vi "Initialize Battle Dialog.vi"() -> (2 "Dashboard":T1[](array[typedef]), 3 "SquareBattle out":refnum<class "SquareBattle Arena.lvclass">, 4 "Intensity Graph Values":cluster{dbl, u32}[](array[cluster]), 6 "Continue?":bool)   [LabVIEW 2014, in "SquareBattle Arena.lvlib" / "SquareBattle Arena.lvclass"]
uses:
  SquareBattle Arena.lvclass
  Dashboard.ctl
  Runner Cluster.ctl
  Square/Square.lvclass
  Square/Square.lvclass/Square.ctl
  SquareBattle Arena.lvclass/SquareBattle Arena.ctl
  Endigit Library/Endigit.lvlib
panel:
  in  "Default Colors":u32[](array[colorbox])=[11163013, 4877194, 13936746, 10864227, 9567230, 16776960, 12868095, 16762130]
  in  "Background Color":u32(colorbox)
  in  "Players":cluster{"Player":u16, "Color":u32}[](array[cluster]) {"Player" items=["Sleepy Engineer"=2, "Line Dancer"=3, "Robert Expand"=7, "Robert Hesitant Wolf"=8, "Robert Hungry Wolf"=9, "Robert Lone Wolf"=10, "Robert Net"=11, "Robert Spawn"=13, "Robert Spread"=14, "Shawn the Explorer"=15, "Shawn the Wanderer"=16]}
  in  "Cancel":bool
  in  "Start":bool
  in  "Board size":i32=150
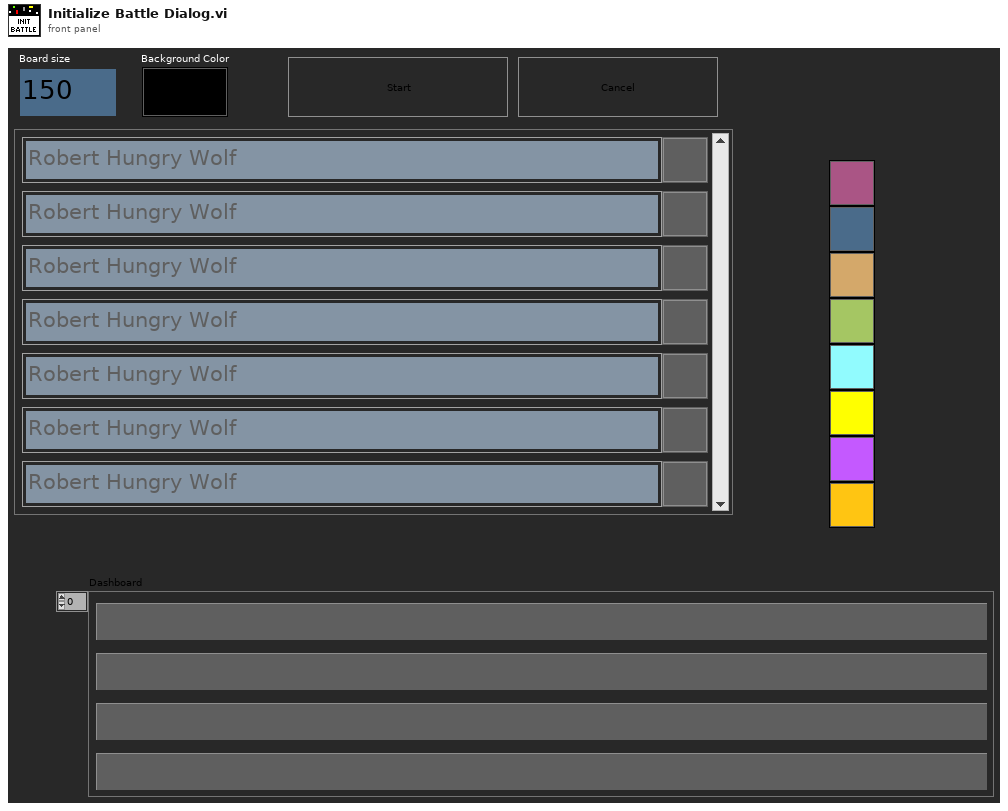
[diagram p1: front panel]
types:
  T1 = typedef "SquareBattle Arena.lvlib/SquareBattle Arena.lvclass/Dashboard.ctl" = cluster{"Color":u32, "Player":string, "Status":string}
  T2 = typedef "SquareBattle Arena.lvlib/SquareBattle Arena.lvclass/Runner Cluster.ctl" = cluster{"Attacked?":bool, "DVR":refnum<data-value>, "Team":i32, "Player":i32, "Next Turn":i32}
  T3 = typedef "SquareBattle Arena.lvlib/SquareBattle Arena.lvclass/Player Info.ctl" = cluster{"Name":string, "Color Box":u32, "Gloat Phrase":string}
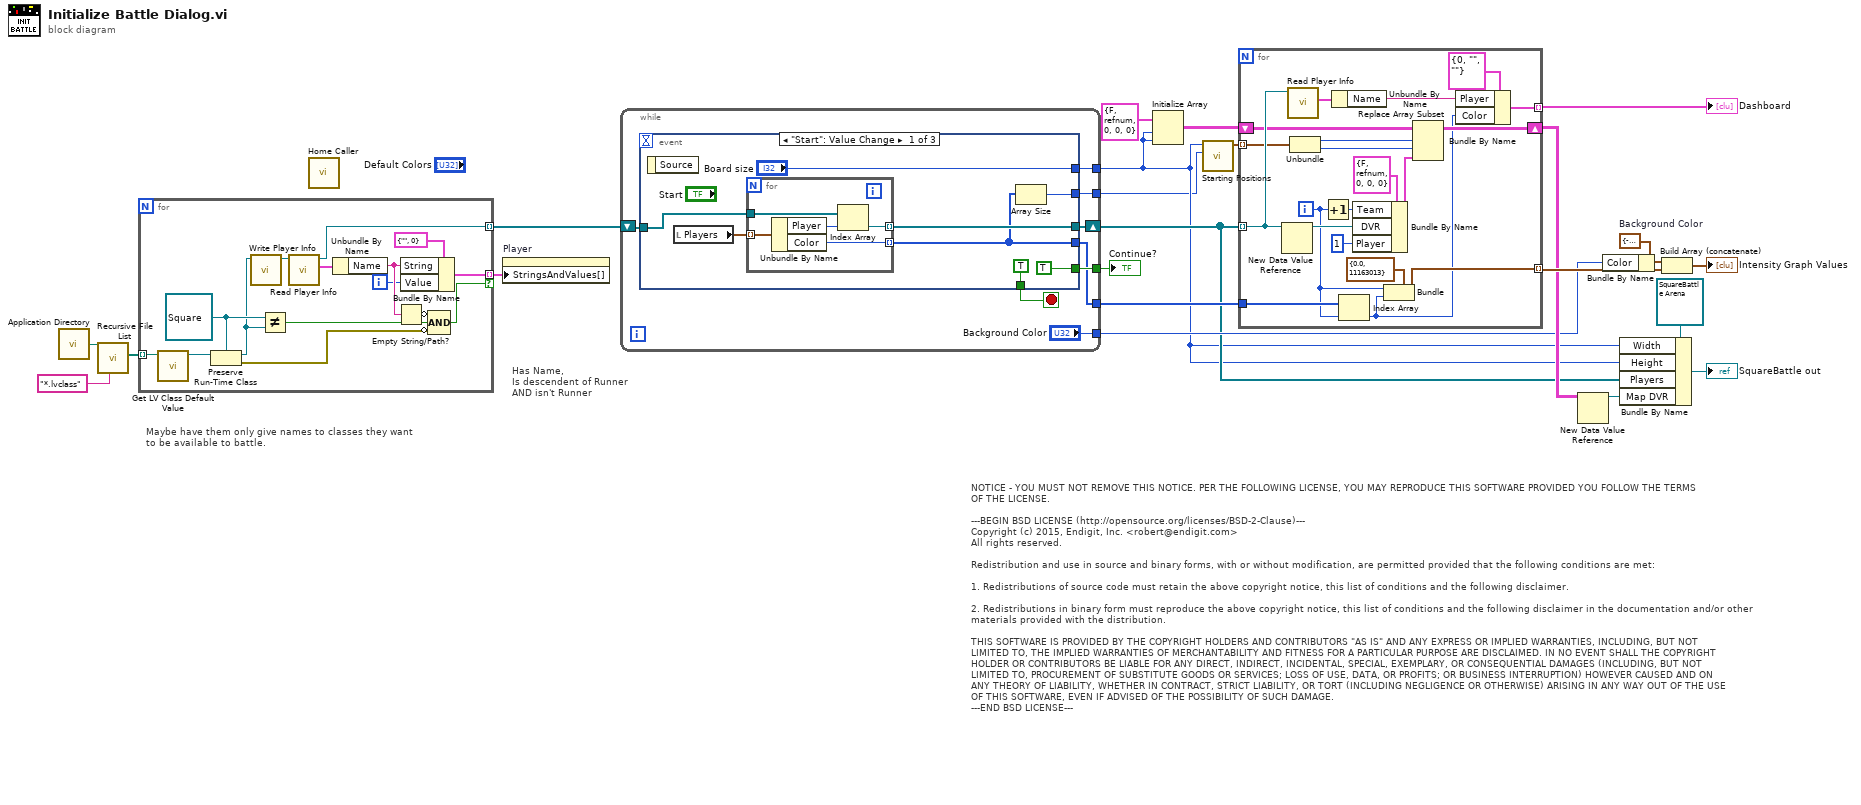
[diagram p0: block diagram]
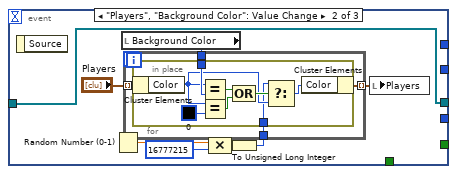
[diagram p2: hidden frame]
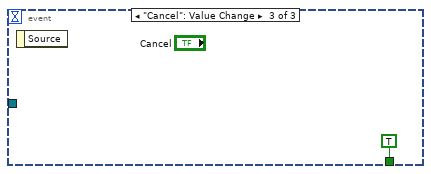
[diagram p3: hidden frame]
diagram:
  w16 = cluster{dbl, "Color":u32} {-1.0, "Color"=16711680}  # Background Color
  # "Has Name,\nIs descendent of Runner\nAND isn't Runner"
  # "NOTICE - YOU MUST NOT REMOVE THIS NOTICE. PER THE FOLLOWING LICENSE, YOU MAY REPRODUCE THIS SOFTWARE PROVIDED YOU FOLLOW THE TERMS\nOF THE LICENSE.\n\n---BEGIN BSD LICENSE (http://opensource.org/licenses/BSD-2-Clause)---\nCopyright (c) 2015, Endigit, Inc. <robert@endigit.com>\nAll rights reserved.\n\nRedistribution and use in source and binary forms, with or without modification, are permitted provided that the following conditions are met:\n\n1. Redistributions of source code must retain the above copyright notice, this list of conditions and the following disclaimer.\n\n2. Redistributions in binary form must reproduce the above copyright notice, this list of conditions and the following disclaimer in the documentation and/or other \nmaterials provided with the distribution.\n\nTHIS SOFTWARE IS PROVIDED BY THE COPYRIGHT HOLDERS AND CONTRIBUTORS \"AS IS\" AND ANY EXPRESS OR IMPLIED WARRANTIES, INCLUDING, BUT NOT \nLIMITED TO, THE IMPLIED WARRANTIES OF MERCHANTABILITY AND FITNESS FOR A PARTICULAR PURPOSE ARE DISCLAIMED. IN NO EVENT SHALL THE COPYRIGHT \nHOLDER OR CONTRIBUTORS BE LIABLE FOR ANY DIRECT, INDIRECT, INCIDENTAL, SPECIAL, EXEMPLARY, OR CONSEQUENTIAL DAMAGES (INCLUDING, BUT NOT \nLIMITED TO, PROCUREMENT OF SUBSTITUTE GOODS OR SERVICES; LOSS OF USE, DATA, OR PROFITS; OR BUSINESS INTERRUPTION) HOWEVER CAUSED AND ON \nANY THEORY OF LIABILITY, WHETHER IN CONTRACT, STRICT LIABILITY, OR TORT (INCLUDING NEGLIGENCE OR OTHERWISE) ARISING IN ANY WAY OUT OF THE USE \nOF THIS SOFTWARE, EVEN IF ADVISED OF THE POSSIBILITY OF SUCH DAMAGE.\n---END BSD LICENSE---"
  # "Maybe have them only give names to classes they want \nto be available to battle."
  n1 = call <vilib>:"Application Directory.vi"() -> ("Application Directory"=w15:path)
  n2 = call <vilib>:"Recursive File List.vi"("pattern"="*.lvclass", "Folder Path"=w15) -> ("All Files in Dir"=w13:path[])  [unwired: 5 in, 4 out]
  n3 = for {
    tunnel: w13 -> [w38] mode=indexing
    tunnel: [w33] -> w8 mode=indexing if=w34
    tunnel: [w31] -> w12 mode=indexing
    i -> [w25]
    w36 = refnum<class "Square.lvclass"> refnum ("Runner.lvclass")
    n4 = call <vilib>:"Get LV Class Default Value.vi"("class path"=w38) -> ("object"=w37:refnum<class>)  [unwired: 9 in, 1 out]
    n5 = Preserve Run-Time Class(object in=w37, 2:w36) -> (object out=w32:refnum<class "Square.lvclass">, error out=w24:errorcluster)  [unwired: 1 in]
    n6 = call-dynamic "Write Player Info.vi"("Runner in"=w32) -> ("Runner out"=w29:refnum<class "Square.lvclass">)  [unwired: 9 in, 1 out]
    n7 = Not Equal?(x=w36, y=w32) -> (x != y?=w35:bool)
    n8 = call "Read Player Info.vi"("Runner in"=w29) -> ("Player Info"=w30:T3, "Runner out"=w31:refnum<class "Square.lvclass">)  [unwired: 8 in, 1 out]
    n9 = Unbundle By Name(w30) -> ("Name"=w28:string)
    n10 = Empty String/Path?(string/path=w28) -> (empty?=w27:bool)
    n11 = Bundle By Name(cluster=cluster{"String":string, "Value":u16} {"String"="", "Value"=0}, "String"=w28, "Value"=w25) -> (w33:cluster{"String":string, "Value":u16})
    n12 = Compound Arithmetic op=AND(invert w27, w35, invert w24) -> (w34:bool)
  }
  n13 = call "Home Caller.vi"() -> ()  [unwired: 11 in]
  n14 = property on="Player" class="Ring (strict)"("StringsAndValues[]"=w8) -> ()  [unwired: 2 in, 2 out]
  n15 = while {
    tunnel: [w46] -> w3
    tunnel: [w45] -> w18
    tunnel: ["Background Color"] -> w10
    tunnel: [w42] -> w9
    shift-right: [w43] -> w4
    shift-left: w12 -> [w44]
    tunnel: [w39] -> w2
    stop <- w41 stop-if-true
    n16 = event shown="[0] \"Start\": Value Change" {
      selector: _ -> [_ _ _]
      dyn-events: _ -> [_ _ _]
      timeout: _ -> [_ _ _]
      tunnel: ["Board size" _ _] -> w46
      tunnel: [TRUE ("Start") _ _] -> w45
      tunnel: w44 -> [w53 w67 _]
      tunnel: [w52 w67 _] -> w43
      tunnel: [w48 _ _] -> w42
      tunnel: [TRUE _ TRUE] -> w41
      tunnel: [w47 _ _] -> w39
      event "Start": Value Change {
        n17 = event-data() -> ()  [unwired: 1 in, 1 out]
        n18 = local read "Players"() -> (w51:cluster{"Player":u16, "Color":u32}[])
        n19 = for {
          tunnel: w51 -> [w58] mode=indexing
          tunnel: w53 -> [w59]
          tunnel: [w57] -> w52 mode=indexing
          tunnel: [w55] -> w48 mode=indexing
          n20 = Unbundle By Name(w58) -> ("Player"=w56:u16, "Color"=w55:u32)
          n21 = Index Array(array=w59, index=w56) -> (element=w57:refnum<class "Square.lvclass">)
        }
        n22 = Array Size(array=w48) -> (size(s)=w47:i32)
      }
      event "Players", "Background Color": Value Change {
        n23 = event-data() -> ()  [unwired: 1 in, 1 out]
        n24 = Random Number (0-1)() -> (number: 0 to 1=w62:dbl)
        n25 = local read "Background Color"() -> (w64:u32)
        n26 = Compound Arithmetic op=MULTIPLY(w62, 16777215) -> (w61:dbl)
        n27 = To Unsigned Long Integer(number=w61) -> (unsigned 32bit integer=w60:u32)
        n28 = for {
          tunnel: "Players" -> [w71] mode=indexing
          tunnel: [w70] -> w65 mode=indexing
          tunnel: w64 -> [w69]
          tunnel: w60 -> [w68]
          n29 = in-place {
            in-place-border: w69 -> [w79]
            in-place-border: w68 -> [w72]
            n30 = in-place-cluster #1(w71) -> ("Color"=w74:u32)
            n31 = Equal?(x=w74, y=w79) -> (x = y?=w77:bool)
            n32 = Equal?(x=w74, y=u32 0) -> (x = y?=w76:bool)
            n33 = Compound Arithmetic op=OR(w77, w76) -> (w75:bool)
            n34 = Select(t=w72, s=w75, f=w74) -> (s? t:f=w73:u32)
            n35 = in-place-cluster #1("Color"=w73) -> (w70:cluster{"Player":u16, "Color":u32})
          }
        }
        n36 = local write "Players"(w65) -> ()
      }
      event "Cancel": Value Change {
        n37 = event-data() -> ()  [unwired: 1 in, 1 out]
      }
    }
  }
  "Continue?" <- w18
  n38 = Initialize Array(T2 {"Attacked?"=FALSE, "DVR"=refnum, "Team"=0, "Player"=0, "Next Turn"=0} ("Cluster"), w3, w3) -> (w6:T2[][])
  n39 = call "Starting Positions.vi"("Player Count"=w2, "Size"=w3) -> ("Positions[]"=w1:cluster{i32, i32}[])  [unwired: 9 in]
  n40 = for {
    tunnel: w4 -> [w89] mode=indexing
    shift-right: [w99] -> w21
    shift-left: w6 -> [w88]
    tunnel: [w93] -> w23 mode=indexing
    tunnel: w9 -> [w92]
    tunnel: [w86] -> w5 mode=indexing
    tunnel: w1 -> [w82] mode=indexing
    i -> [w90]
    n41 = New Data Value Reference(data value=w89) -> (data value reference=w98:refnum<data-value>)  [unwired: 1 in, 1 out]
    n42 = call "Read Player Info.vi"("Runner in"=w89) -> ("Player Info"=w96:T3)  [unwired: 8 in, 2 out]
    n43 = Unbundle(w82) -> (w83:i32, w81:i32)
    n44 = Increment(x=w90) -> (x+1=w85:i32)
    n45 = Unbundle By Name(w96) -> ("Name"=w95:string)
    n46 = Index Array(array=w92, index=w90) -> (element=w91:u32)
    n47 = Bundle By Name(cluster=T2 {"Attacked?"=FALSE, "DVR"=refnum, "Team"=0, "Player"=0, "Next Turn"=0} ("Cluster"), "Team"=w85, "DVR"=w98, "Player"=1) -> (w87:T2)
    n48 = Bundle(cluster=cluster{dbl, u32} {0.0, 11163013}, w90, w91) -> (w93:cluster{dbl, u32})
    n49 = Replace Array Subset(array=w88, new element=w87, index (row)=w83, index (col)=w81) -> (w99:T2[][])
    n50 = Bundle By Name(cluster=T1 {"Color"=0, "Player"="", "Status"=""} ("Dashboard"), "Player"=w95, "Color"=w91) -> (w86:T1)
  }
  "Dashboard" <- w5
  n51 = New Data Value Reference(data value=w21) -> (data value reference=w20:refnum<data-value>)  [unwired: 1 in, 1 out]
  n52 = Bundle By Name(cluster=w16, "Color"=w10) -> (w11:cluster{dbl, "Color":u32})
  n53 = Bundle By Name(cluster=refnum<class "SquareBattle Arena.lvclass"> refnum ("Maze 2.0.lvclass"), "Width"=w3, "Height"=w3, "Players"=w4, "Map DVR"=w20) -> (→"SquareBattle out":refnum<class "SquareBattle Arena.lvclass">)
  n54 = Build Array (concatenate)(w11, w23) -> (→"Intensity Graph Values":cluster{dbl, "Color":u32}[])
